vi "setup_lc_tg.vi"(0 "shuoming":string, 1 "didian":string, 4 "zhriqi":string, 6 "jsren":string, 9 "yw":string, 10 "id":string, 11 "zc_luodi_num":string) -> (2 "error":errorcluster caption="error out 2")   [LabVIEW 2017, in "Lib_code.lvlib"]
uses:
  Lib_code.lvlib
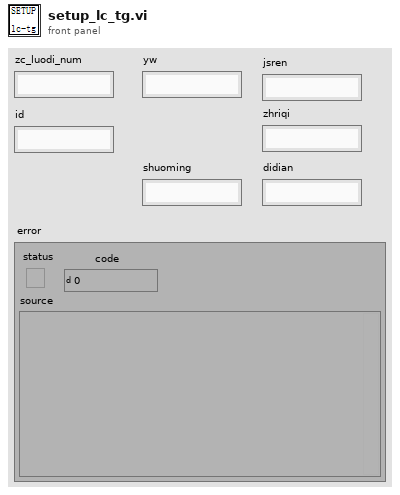
[diagram p1: front panel]
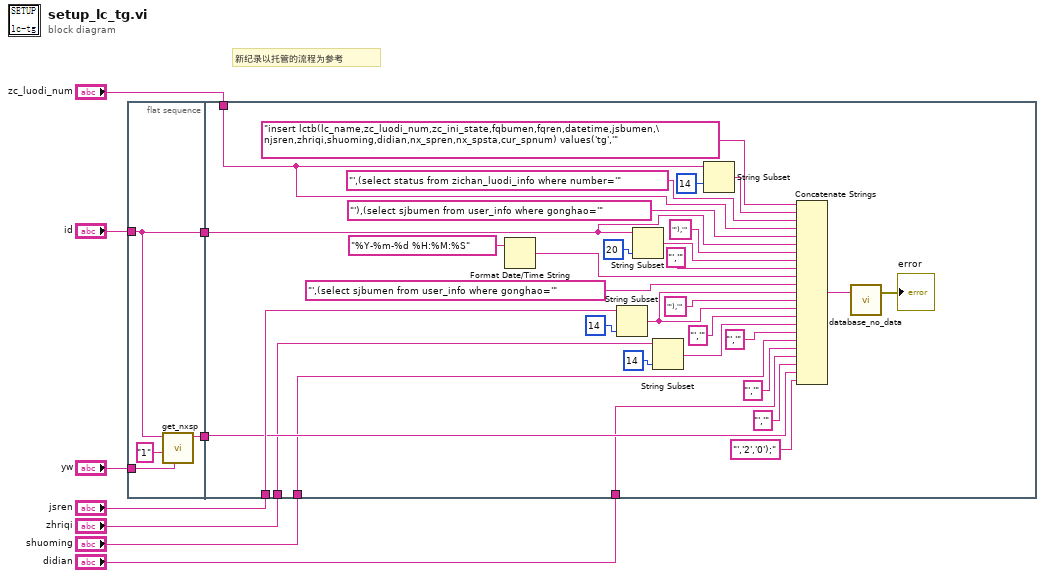
[diagram p0: block diagram]
diagram:
  # "新纪录以托管的流程为参考"
  n1 = flat-sequence {
    tunnel: "id" -> [w12]
    tunnel: [w12] -> w8
    tunnel: [w13] -> w7
    tunnel: "yw" -> [w11]
    tunnel: w8 -> [w23]
    tunnel: w7 -> [w33]
    tunnel: "zc_luodi_num" -> [w25]
    tunnel: "jsren" -> [w34]
    tunnel: "shuoming" -> [w19]
    tunnel: "didian" -> [w30]
    tunnel: "zhriqi" -> [w27]
    frame #0 {
      n2 = call "get_nxsp.vi"("yw"=w11, "Cur_state"="1", "fqren"=w12) -> ("sp_gonghao"=w13:string)  [unwired: 6 in, 2 out]
    }
    frame #1 {
      n3 = Format Date/Time String(time format string (%c)="%Y-%m-%d %H:%M:%S" ("时间格式字符串(%c)")) -> (date/time string=w17:string)  [unwired: 2 in]
      n4 = String Subset(string=w34, length (rest)=14 ("长度（剩余）")) -> (substring=w15:string)  [unwired: 1 in]
      n5 = String Subset(string=w23, length (rest)=20 ("长度（剩余）")) -> (substring=w37:string)  [unwired: 1 in]
      n6 = String Subset(string=w27, length (rest)=14 ("长度（剩余）")) -> (substring=w18:string)  [unwired: 1 in]
      n7 = String Subset(string=w25, length (rest)=14 ("长度（剩余）")) -> (substring=w42:string)  [unwired: 1 in]
      n8 = Concatenate Strings("insert lctb(lc_name,zc_luodi_num,zc_ini_state,fqbumen,fqren,datetime,jsbumen,\njsren,zhriqi,shuoming,didian,nx_spren,nx_spsta,cur_spnum) values('tg','" ("格式字符串"), w42, "',(select status from zichan_luodi_info where number='" ("字符串"), w25, "'),(select sjbumen from user_info where gonghao='" ("字符串"), w23, "'),'" ("字符串"), w37, "','" ("字符串"), w17, "',(select sjbumen from user_info where gonghao='" ("字符串"), w15, "'),'" ("字符串"), w15, "','" ("字符串"), w18, "','" ("字符串"), w19, "','" ("字符串"), w30, "','" ("字符串"), w33, "','2','0');" ("字符串")) -> (w32:string)
      n9 = call "database_no_data.vi"("input"=w32) -> ("error"=→"error":errorcluster)  [unwired: 2 in]
    }
  }
